vi "Configure ALC.vi"(0 "VISA resource name":refnum<visa-resource-name>, 1 "Enable ALC (T:Enable)":bool=TRUE, 5 "ALC Level (1 dB)":dbl=1.0, 7 "Enable Automatic Bandwidth (T:Enable)":bool=TRUE, 9 "ALC Bandwidth (0: 100 Hz)":u16(ring) items=["100 Hz", "1 kHz", "10 kHz", "100 kHz", "200 Hz", "2 kHz", "20 kHz"], 11 "error in (no error)":errorcluster, 12 "ALC Source (0: Internal)":u16(ring) items=["Internal", "External Detector", "Millimeter-wave"], 13 "External Detector Coupling Factor (16 dB)":dbl=16.0) -> (4 "VISA resource name out":refnum<visa-resource-name>, 15 "error out":errorcluster)   [LabVIEW 2012, in "Agilent PSG MXG Series.lvlib"]
doc: "Configures ALC (automatic leveling control) state, ALC level, ALC bandwidth, and ALC source of the signal generator."
uses:
  <instrlib>/Agilent PSG MXG Series/Agilent PSG MXG Series.lvlib
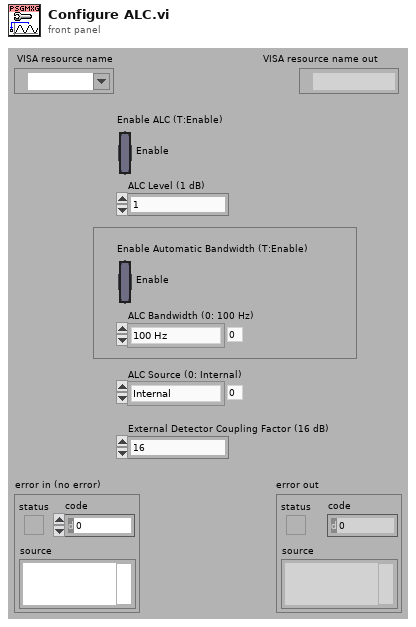
[diagram p1: front panel]
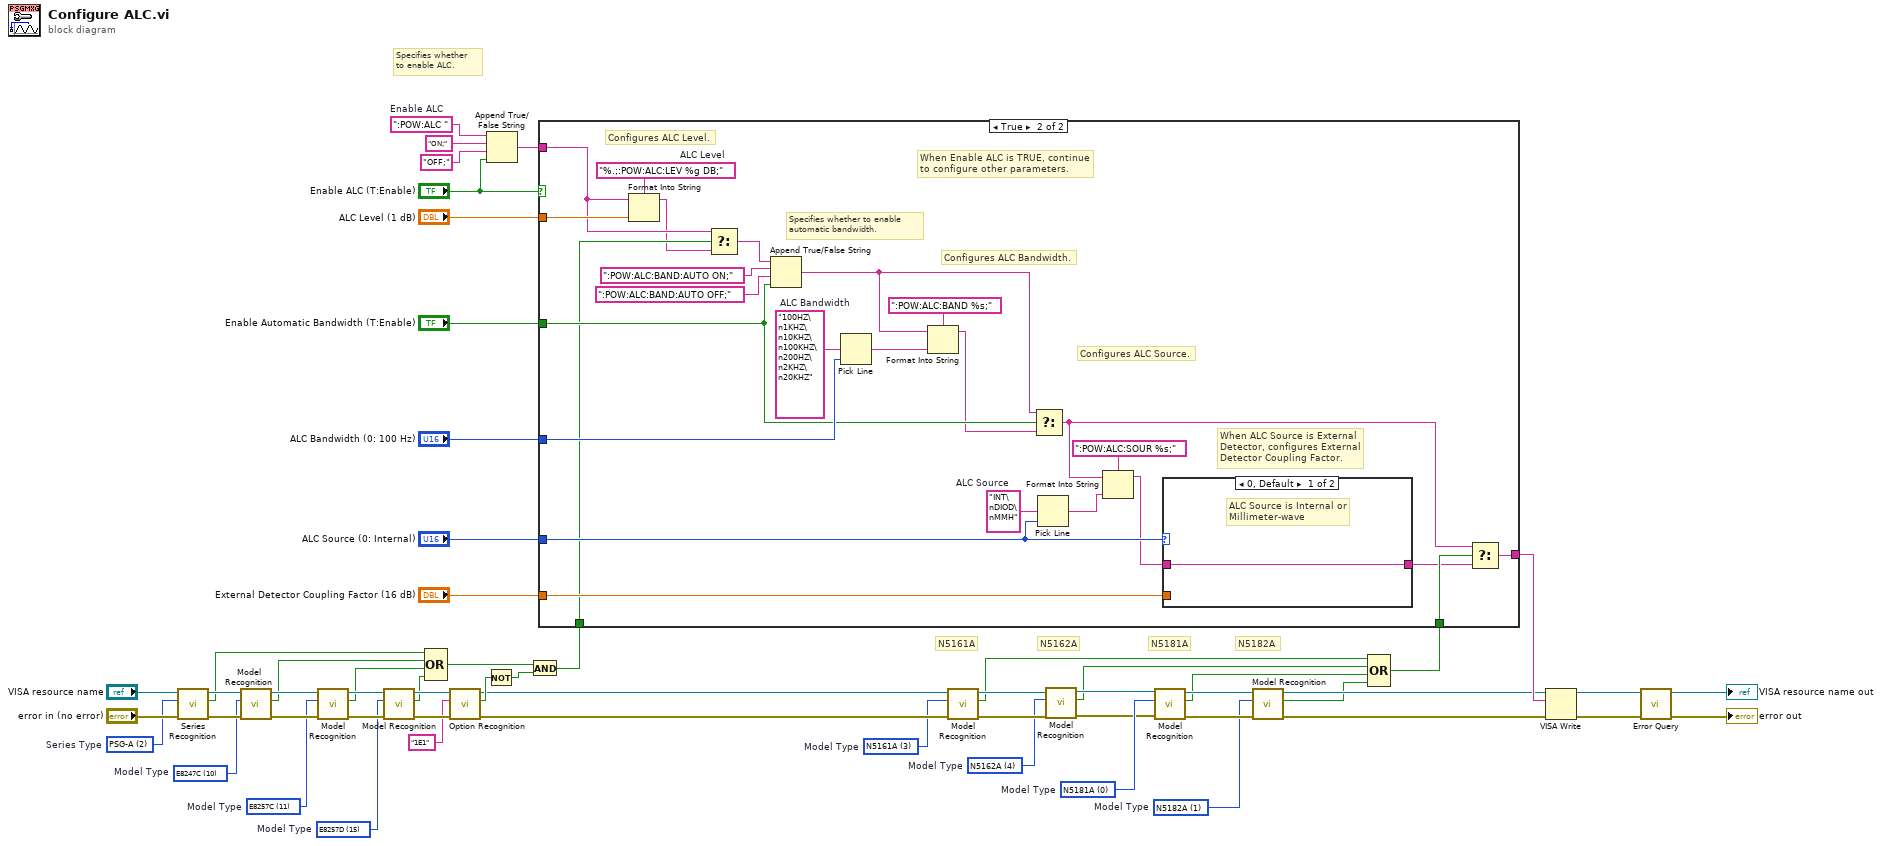
[diagram p0: block diagram]
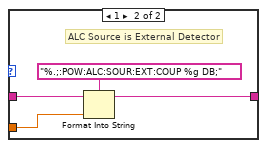
[diagram p3: hidden frame]
diagram:
  w6 = u16 3 items=["N5181A"=0, "N5182A"=1, "N5183A"=2, "N5161A"=3, "N5162A"=4, "E8241A"=5, "E8244A"=6, "E8251A"=7, "E8254A"=8, "E8247C"=10, "E8257C"=11, "E8267C"=12, "E8257D"=15, "E8267D"=16, "N5171B"=17, "N5172B"=18, "N5181B"=19, "N5182B"=20]  # Model Type
  w7 = u16 4 items=["N5181A"=0, "N5182A"=1, "N5183A"=2, "N5161A"=3, "N5162A"=4, "E8241A"=5, "E8244A"=6, "E8251A"=7, "E8254A"=8, "E8247C"=10, "E8257C"=11, "E8267C"=12, "E8257D"=15, "E8267D"=16, "N5171B"=17, "N5172B"=18, "N5181B"=19, "N5182B"=20]  # Model Type
  w14 = u16 1 items=["N5181A"=0, "N5182A"=1, "N5183A"=2, "N5161A"=3, "N5162A"=4, "E8241A"=5, "E8244A"=6, "E8251A"=7, "E8254A"=8, "E8247C"=10, "E8257C"=11, "E8267C"=12, "E8257D"=15, "E8267D"=16, "N5171B"=17, "N5172B"=18, "N5181B"=19, "N5182B"=20]  # Model Type
  w15 = u16 0 items=["N5181A"=0, "N5182A"=1, "N5183A"=2, "N5161A"=3, "N5162A"=4, "E8241A"=5, "E8244A"=6, "E8251A"=7, "E8254A"=8, "E8247C"=10, "E8257C"=11, "E8267C"=12, "E8257D"=15, "E8267D"=16, "N5171B"=17, "N5172B"=18, "N5181B"=19, "N5182B"=20]  # Model Type
  w16 = u16 2 items=["MXG-A", "PSG", "PSG-A", "PSG-C", "PSG-D", "MXG-B", "EXG"]  # Series Type
  w17 = u16 10 items=["N5181A"=0, "N5182A"=1, "N5183A"=2, "N5161A"=3, "N5162A"=4, "E8241A"=5, "E8244A"=6, "E8251A"=7, "E8254A"=8, "E8247C"=10, "E8257C"=11, "E8267C"=12, "E8257D"=15, "E8267D"=16, "N5171B"=17, "N5172B"=18, "N5181B"=19, "N5182B"=20]  # Model Type
  w18 = u16 11 items=["N5181A"=0, "N5182A"=1, "N5183A"=2, "N5161A"=3, "N5162A"=4, "E8241A"=5, "E8244A"=6, "E8251A"=7, "E8254A"=8, "E8247C"=10, "E8257C"=11, "E8267C"=12, "E8257D"=15, "E8267D"=16, "N5171B"=17, "N5172B"=18, "N5181B"=19, "N5182B"=20]  # Model Type
  w19 = u16 15 items=["N5181A"=0, "N5182A"=1, "N5183A"=2, "N5161A"=3, "N5162A"=4, "E8241A"=5, "E8244A"=6, "E8251A"=7, "E8254A"=8, "E8247C"=10, "E8257C"=11, "E8267C"=12, "E8257D"=15, "E8267D"=16, "N5171B"=17, "N5172B"=18, "N5181B"=19, "N5182B"=20]  # Model Type
  w57 = ":POW:ALC "  # Enable ALC
  # "N5161A"
  # "N5162A"
  # "N5181A"
  # "N5182A"
  # "Specifies whether\nto enable ALC."
  n1 = call <instrlib>:"Series Recognition.vi"("error in (no error)"="error in (no error)", "Series Type (0: MXG)"=w16, "VISA resource name"="VISA resource name") -> ("error out"=w35:errorcluster, "Is Series Correct"=w27:bool, "VISA resource name out"=w36:refnum<visa-resource-name>)  [unwired: 6 out]
  n2 = call <instrlib>:"Model Recognition.vi"("error in (no error)"=w35, "Model Type (0: N5181A)"=w17, "VISA resource name"=w36) -> ("error out"=w33:errorcluster, "Is Model Correct"=w26:bool, "VISA resource name out"=w34:refnum<visa-resource-name>)  [unwired: 6 out]
  n3 = call <instrlib>:"Model Recognition.vi"("error in (no error)"=w33, "Model Type (0: N5181A)"=w18, "VISA resource name"=w34) -> ("error out"=w31:errorcluster, "Is Model Correct"=w25:bool, "VISA resource name out"=w32:refnum<visa-resource-name>)  [unwired: 6 out]
  n4 = call <instrlib>:"Model Recognition.vi"("error in (no error)"=w31, "Model Type (0: N5181A)"=w19, "VISA resource name"=w32) -> ("error out"=w29:errorcluster, "Is Model Correct"=w24:bool, "VISA resource name out"=w30:refnum<visa-resource-name>)  [unwired: 6 out]
  n5 = Compound Arithmetic op=OR(w27, w26, w25, w24) -> (w22:bool)
  n6 = call <instrlib>:"Option Recognition.vi"("error in (no error)"=w29, "Option (\"\")"="1E1" ("Option (\"\")"), "VISA resource name"=w30) -> ("error out"=w8:errorcluster, "Is Option Installed"=w23:bool, "VISA resource name out"=w9:refnum<visa-resource-name>)  [unwired: 6 out]
  n7 = Not(x=w23) -> (.not. x?=w21:bool)
  n8 = Append True/False String(1:"Enable ALC (T:Enable)", 2:"OFF;" ("false string"), 3:"ON;" ("true string"), 4:w57) -> (0:w55:string)
  n9 = And(x=w22, y=w21) -> (x .and. y?=w20:bool)
  n10 = call <instrlib>:"Model Recognition.vi"("error in (no error)"=w8, "Model Type (0: N5181A)"=w6, "VISA resource name"=w9) -> ("error out"=w11:errorcluster, "Is Model Correct"=w2:bool, "VISA resource name out"=w13:refnum<visa-resource-name>)  [unwired: 6 out]
  n11 = call <instrlib>:"Model Recognition.vi"("error in (no error)"=w11, "Model Type (0: N5181A)"=w7, "VISA resource name"=w13) -> ("error out"=w10:errorcluster, "Is Model Correct"=w3:bool, "VISA resource name out"=w12:refnum<visa-resource-name>)  [unwired: 6 out]
  n12 = call <instrlib>:"Model Recognition.vi"("error in (no error)"=w10, "Model Type (0: N5181A)"=w15, "VISA resource name"=w12) -> ("error out"=w41:errorcluster, "Is Model Correct"=w4:bool, "VISA resource name out"=w42:refnum<visa-resource-name>)  [unwired: 6 out]
  n13 = call <instrlib>:"Model Recognition.vi"("error in (no error)"=w41, "Model Type (0: N5181A)"=w14, "VISA resource name"=w42) -> ("error out"=w39:errorcluster, "Is Model Correct"=w5:bool, "VISA resource name out"=w40:refnum<visa-resource-name>)  [unwired: 6 out]
  n14 = Compound Arithmetic op=OR(w2, w3, w4, w5) -> (w1:bool)
  n15 = case shown="True" "Enable ALC (T:Enable)" {
    tunnel: w55 -> [w58 w61]
    tunnel: "ALC Level (1 dB)" -> [_ w83]
    tunnel: "ALC Bandwidth (0: 100 Hz)" -> [_ w78]
    tunnel: "Enable Automatic Bandwidth (T:Enable)" -> [_ w76]
    tunnel: "ALC Source (0: Internal)" -> [_ w66]
    tunnel: "External Detector Coupling Factor (16 dB)" -> [_ w67]
    tunnel: [w58 w70] -> w48
    tunnel: w1 -> [_ w68]
    tunnel: w20 -> [_ w62]
    frame False {
      # "When Enable ALC\nis FALSE, do nothing."
    }
    frame True {
      w71 = "INT\nDIOD\nMMH"  # ALC Source
      w79 = "100HZ\n1KHZ\n10KHZ\n100KHZ\n200HZ\n2KHZ\n20KHZ"  # ALC Bandwidth
      w82 = "%.;:POW:ALC:LEV %g DB;"  # ALC Level
      # "When ALC Source is External\nDetector, configures External\nDetector Coupling Factor."
      # "Configures ALC Source."
      # "Configures ALC Bandwidth."
      # "Specifies whether to enable\nautomatic bandwidth."
      # "Configures ALC Level."
      # "When Enable ALC is TRUE, continue\nto configure other parameters."
      n16 = Format Into String(format string=w82, initial string=w61, w83) -> (resulting string=w60:string)  [unwired: 1 in, 1 out]
      n17 = Select(t=w61, s=w62, f=w60) -> (s? t:f=w59:string)
      n18 = Append True/False String(1:w76, 2:":POW:ALC:BAND:AUTO OFF;" ("format string"), 3:":POW:ALC:BAND:AUTO ON;" ("format string"), 4:w59) -> (0:w75:string)
      n19 = Pick Line(multi-line string=w79, line index=w78) -> (output string=w77:string)  [unwired: 1 out]
      n20 = Format Into String(format string=":POW:ALC:BAND %s;", initial string=w75, w77) -> (resulting string=w74:string)  [unwired: 1 in, 1 out]
      n21 = Select(t=w75, s=w76, f=w74) -> (s? t:f=w69:string)
      n22 = Pick Line(multi-line string=w71, line index=w66) -> (output string=w72:string)  [unwired: 1 out]
      n23 = Format Into String(format string=":POW:ALC:SOUR %s;", initial string=w69, w72) -> (resulting string=w64:string)  [unwired: 1 in, 1 out]
      n24 = case shown="0, Default" w66 {
        tunnel: w67 -> [_ w87]
        tunnel: [w84 w86] -> w65
        tunnel: w64 -> [w84 w85]
        frame 0, Default {
          # "ALC Source is Internal or\nMillimeter-wave"
        }
        frame 1 {
          # "ALC Source is External Detector"
          n25 = Format Into String(format string="%.;:POW:ALC:SOUR:EXT:COUP %g DB;", initial string=w85, w87) -> (resulting string=w86:string)  [unwired: 1 in, 1 out]
        }
      }
      n26 = Select(t=w69, s=w68, f=w65) -> (s? t:f=w70:string)
    }
  }
  n27 = VISA Write(VISA resource name=w40, write buffer=w48, error in (no error)=w39) -> (VISA resource name out=w47:refnum<visa-resource-name>, error out=w46:errorcluster)  [unwired: 1 out]
  n28 = call <instrlib>:"Error Query.vi"("error in (no error)"=w46, "VISA resource name"=w47) -> ("error out"=→"error out":errorcluster, "VISA resource name out"=→"VISA resource name out":refnum<visa-resource-name>)  [unwired: 8 out]
